vi "Get Constants.vi"() -> (3 "Constants":cluster{"name":string, "value":dbl}[](array[cluster]))   [LabVIEW 2024, in "Output Sequencer.lvlib" / "Output Sequencer.lvclass"]
uses:
  Output Sequencer.lvclass
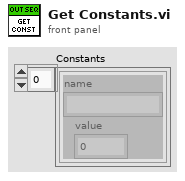
[diagram p1: front panel]
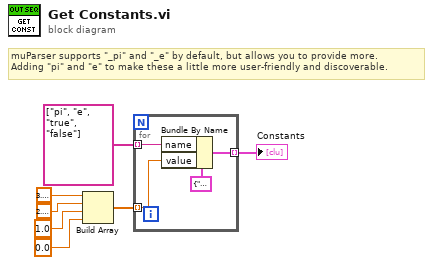
[diagram p0: block diagram]
diagram:
  # "muParser supports \"_pi\" and \"_e\" by default, but allows you to provide more.\nAdding \"pi\" and \"e\" to make these a little more user-friendly and discoverable."
  n1 = Build Array(3.141592653589793, 2.718281828459045, 1.0, 0.0) -> (w2:dbl[])
  n2 = for {
    tunnel: string[] ["pi", "e", "true", "false"] -> [w10] mode=indexing
    tunnel: w2 -> [w9] mode=indexing
    tunnel: [w8] -> w1 mode=indexing
    n3 = Bundle By Name(cluster=cluster{"name":string, "value":dbl} {"name"="", "value"=0.0} ("Cluster"), "name"=w10, "value"=w9) -> (w8:cluster{"name":string, "value":dbl})
  }
  "Constants" <- w1
